vi "CreateWO-RequiredFieldsMissing.vi"(8 "error in":errorcluster, 11 "ERP-CreateWorkOrder in":refnum<class "ERP-CreateWorkOrder.lvclass">) -> (0 "error out":errorcluster, 3 "ERP-CreateWorkOrder out":refnum<class "ERP-CreateWorkOrder.lvclass">)   [LabVIEW 2013, in "ERP-CreateWorkOrder.lvclass"]
uses:
  ERP-CreateWorkOrder.lvclass
  ERP-CreateWorkOrder.lvclass/ERP-CreateWorkOrder.ctl
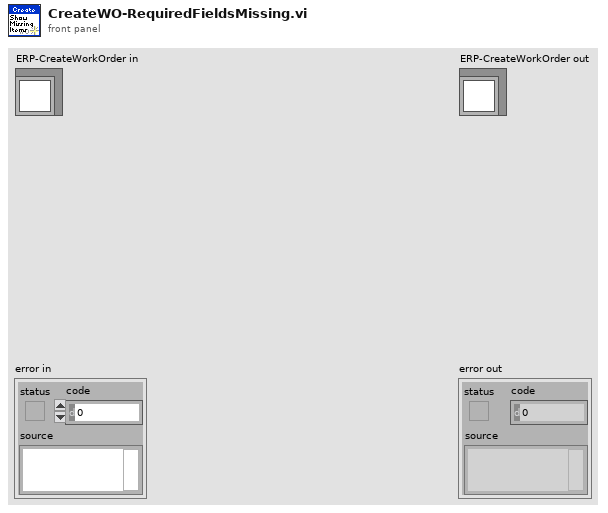
[diagram p1: front panel]
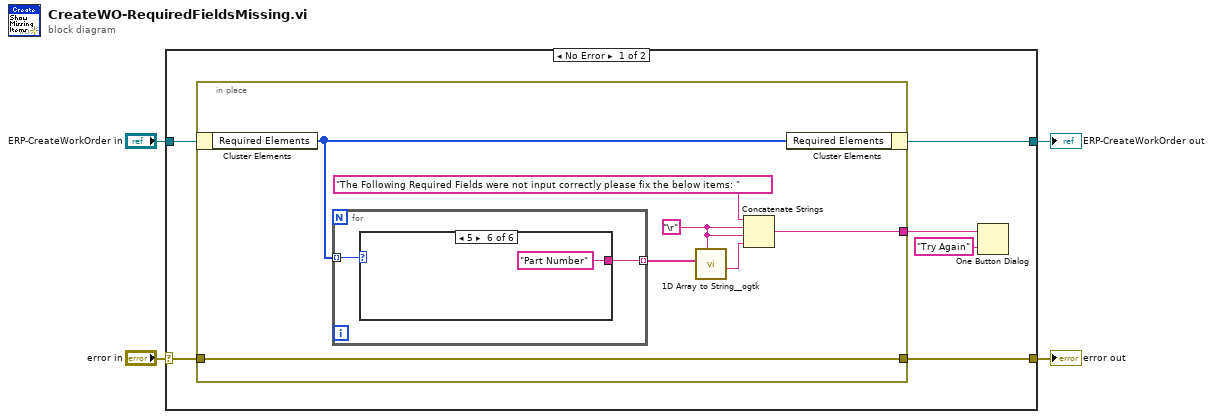
[diagram p0: block diagram]
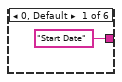
[diagram p2: hidden frame]
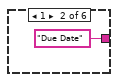
[diagram p3: hidden frame]
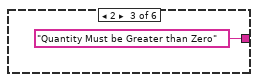
[diagram p4: hidden frame]
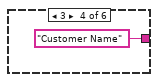
[diagram p5: hidden frame]
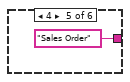
[diagram p6: hidden frame]
diagram:
  n1 = case shown="No Error" "error in" {
    selector: "error in" -> [w10 w27]
    tunnel: [w9 w27] -> w3
    tunnel: [w7 w26] -> w1
    tunnel: "ERP-CreateWorkOrder in" -> [w8 w26]
    frame No Error {
      n2 = in-place {
        in-place-border: w10 -> [w12]
        in-place-border: [w12] -> w9
        in-place-border: [w11] -> w5
        w15 = "\r"
        n3 = in-place-cluster #1(w8) -> ("Required Elements"=w13:i32[])
        n4 = for {
          tunnel: w13 -> [w19] mode=indexing
          tunnel: [w18] -> w14 mode=indexing
          n5 = case shown="5" w19 {
            tunnel: ["Start Date" "Due Date" "Quantity Must be Greater than Zero" "Customer Name" "Sales Order" "Part Number"] -> w18
            frame 0, Default {
            }
            frame 1 {
            }
            frame 2 {
            }
            frame 3 {
            }
            frame 4 {
            }
            frame 5 {
            }
          }
        }
        n6 = call <userlib>:"1D Array to String__ogtk.vi"("delimiter (Tab)"=w15, "Array of Strings"=w14) -> ("delimited string"=w16:string)  [unwired: 9 in]
        n7 = Concatenate Strings("The Following Required Fields were not input correctly please fix the below items: " ("string"), w15, w15, w16) -> (w11:string)
        n8 = in-place-cluster #1("Required Elements"=w13) -> (w7:refnum<class "ERP-CreateWorkOrder.lvclass">)
      }
      n9 = One Button Dialog(message=w5, button name ("OK")="Try Again") -> ()  [unwired: 1 out]
    }
    frame Error {
    }
  }
  "error out" <- w3
  "ERP-CreateWorkOrder out" <- w1
